vi "树控件内置拖动功能.vi"() -> ()   [LabVIEW 2012, in "Tree Tools.lvlib"]
uses:
  Tree Tools.lvlib
panel:
  in  "停止":bool
  in  "已选择人物放置":i32(listbox)
  in  "选择人物拖动":string(tree)="猪八戒_1"
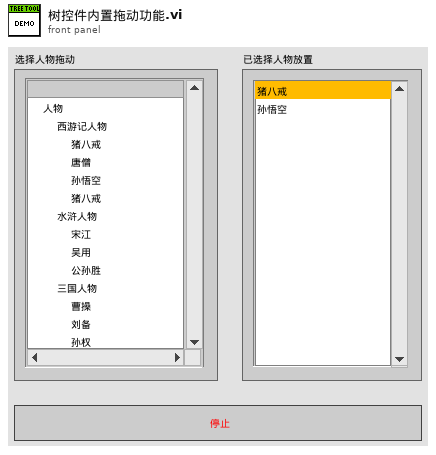
[diagram p1: front panel]
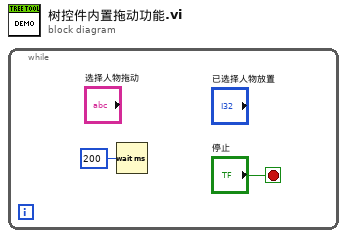
[diagram p0: block diagram]
diagram:
  n1 = while {
    stop <- "停止" stop-if-true
    n2 = Wait (ms)(milliseconds to wait=u32 200 ("等待时间（毫秒）")) -> ()  [unwired: 1 out]
  }
